vi "BSON_bytes_to_bool.vi"(11 "BSONbytes":u8[](array[numeric])) -> (3 "value":bool)   [LabVIEW 2015, in "BSON_convertors_Library.lvlib"]
uses:
  BSON_convertors_Library.lvlib
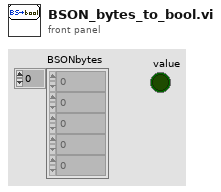
[diagram p1: front panel]
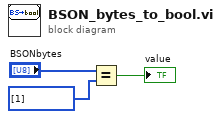
[diagram p0: block diagram]
diagram:
  n1 = Equal?(x="BSONbytes", y=u8[] [1] ("BSONbytes")) -> (x = y?=→"value":bool)
